vi "Set Error.vi"(8 "error in (no error)":errorcluster, 10 "error":errorcluster, 11 "Output Actor Hardware in":refnum<class "Output Actor Hardware.lvclass">) -> (0 "error out":errorcluster, 3 "Output Actor Hardware out":refnum<class "Output Actor Hardware.lvclass">)   [LabVIEW 2015, in "Output Actor Hardware.lvclass"]
uses:
  Output Actor Hardware.lvclass
  Output Actor Hardware.lvclass/Output Actor Hardware.ctl
  output actor/Output Actor.lvclass
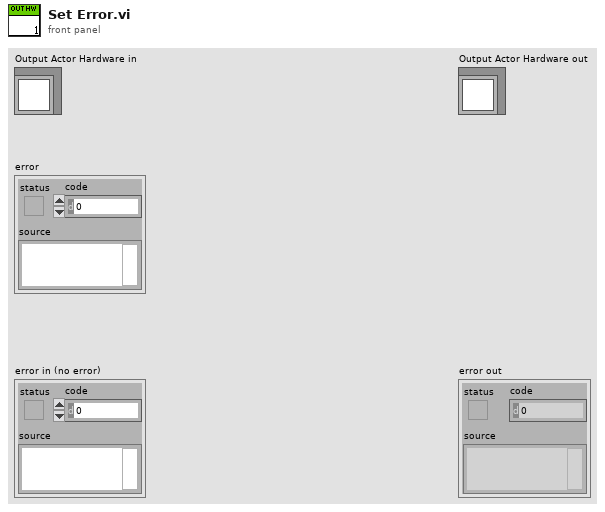
[diagram p1: front panel]
types:
  T1 = cluster{"status":bool, "code":bool, "source":bool}
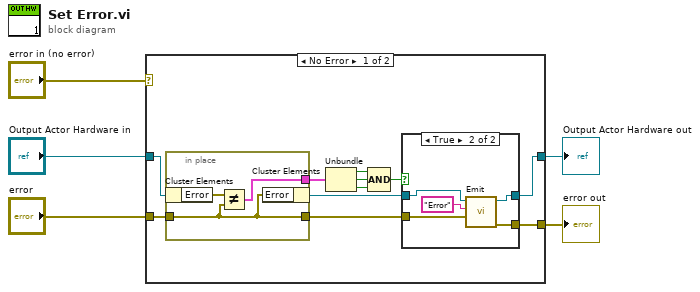
[diagram p0: block diagram]
diagram:
  n1 = case shown="No Error" "error in (no error)" {
    selector: "error in (no error)" -> [_ w27]
    tunnel: [w6 w27] -> w4
    tunnel: [w7 w26] -> w2
    tunnel: "Output Actor Hardware in" -> [w16 w26]
    tunnel: "error" -> [w15 _]
    frame No Error {
      n2 = in-place {
        in-place-border: w15 -> [w23]
        in-place-border: [w24] -> w9
        in-place-border: [w23] -> w14
        n3 = in-place-cluster #1(w16) -> ("Error"=w25:errorcluster)
        n4 = Not Equal?(x=w25, y=w23) -> (x != y?=w24:T1)
        n5 = in-place-cluster #1("Error"=w23) -> (w13:refnum<class "Output Actor Hardware.lvclass">)
      }
      n6 = Unbundle(w9) -> ("status"=w12:bool, "code"=w11:bool, "source"=w10:bool)
      n7 = Compound Arithmetic op=AND(w12, w11, w10) -> (w8:bool)
      n8 = case shown="True" w8 {
        tunnel: w14 -> [_ w21]
        tunnel: w13 -> [w17 w20]
        tunnel: [w17 w18] -> w7
        tunnel: [_ w19] -> w6
        frame False {
        }
        frame True {
          n9 = call "Emit.vi"("parameter"=w21, "function"="Error", "output_actor in"=w20) -> ("error out"=w19:errorcluster, "output_actor out"=w18:refnum<class "Output Actor Hardware.lvclass">)  [unwired: 7 in]
        }
      }
    }
    frame Error {
    }
  }
  "error out" <- w4
  "Output Actor Hardware out" <- w2
